vi "LogLastPortGlobal.vi"(7 "Action":T1, 11 "Set Value":bool[](array[boolean])) -> (3 "Value Out":bool[](array[boolean]))   [LabVIEW 2013]
uses:
  LogLastPortGlobalAction.ctl
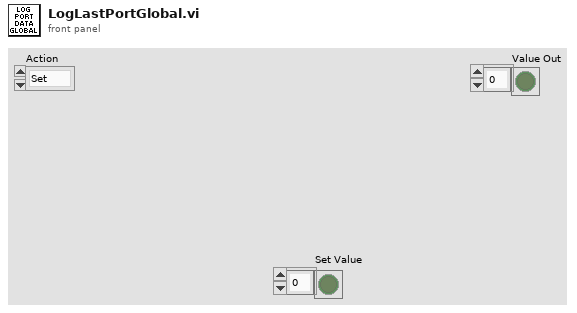
[diagram p1: front panel]
types:
  T1 = typedef "LogLastPortGlobalAction.ctl" = enum16{"Set", "Get"}
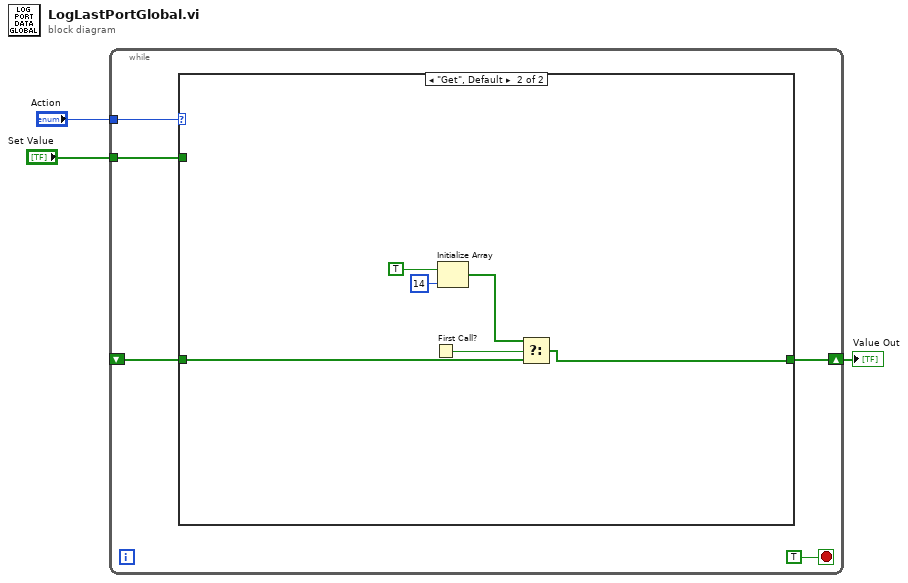
[diagram p0: block diagram]
diagram:
  n1 = while {
    tunnel: "Action" -> [w7]
    tunnel: "Set Value" -> [w6]
    shift-right: [w5] -> w1
    shift-left: _ -> [w4]
    stop <- TRUE stop-if-true
    n2 = case shown="\"Get\", Default" w7 {
      tunnel: w6 -> [w9 _]
      tunnel: [w9 w13] -> w5
      tunnel: w4 -> [_ w14]
      frame "Set" {
      }
      frame "Get", Default {
        n3 = First Call?() -> (First Call?: T/F=w15:bool)
        n4 = Initialize Array(TRUE, 14 ("dimension size")) -> (w10:bool[])
        n5 = Select(t=w10, s=w15, f=w14) -> (s? t:f=w13:bool[])
      }
    }
  }
  "Value Out" <- w1
